vi "Generate Z stage Position Aarray.vi"(5 "Save PSOCT?":bool[](array[boolean]), 7 "#cycles":u32, 8 "Error in":errorcluster, 9 "Pause?":bool[](array[boolean]), 10 "image thickness":u32[](array[numeric]), 11 "slice thickness":u32[](array[numeric])) -> (0 "Error out":errorcluster, 1 "Cut Pauser":bool[](array[boolean]), 2 "image height out":dbl[](array[numeric]), 3 "cut height out":dbl[](array[numeric]), 4 "Save PSOCT?":bool[](array[boolean]))   [LabVIEW 2018]
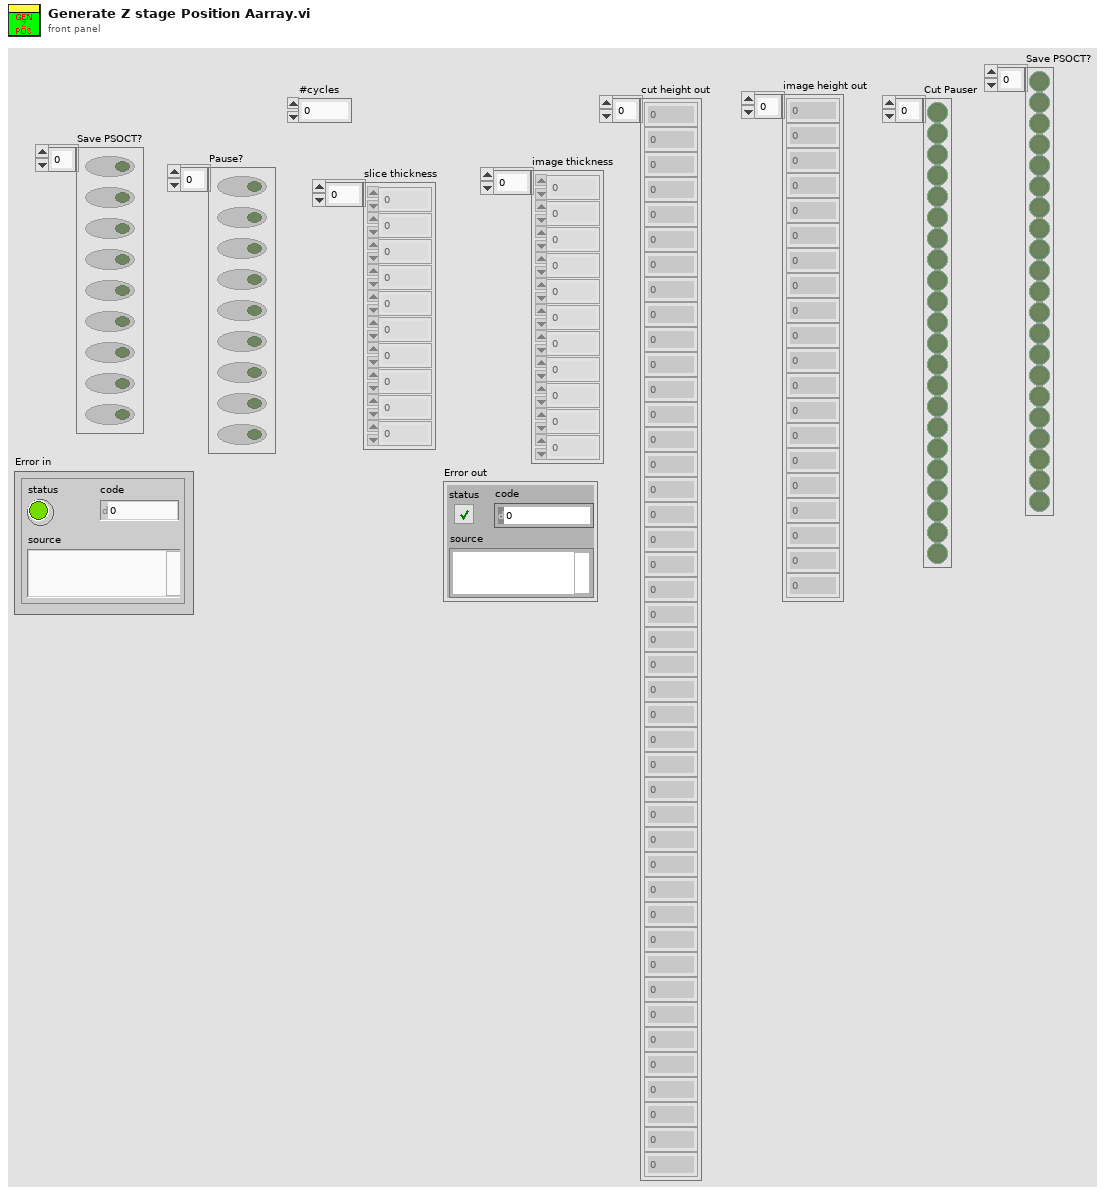
[diagram p1: front panel]
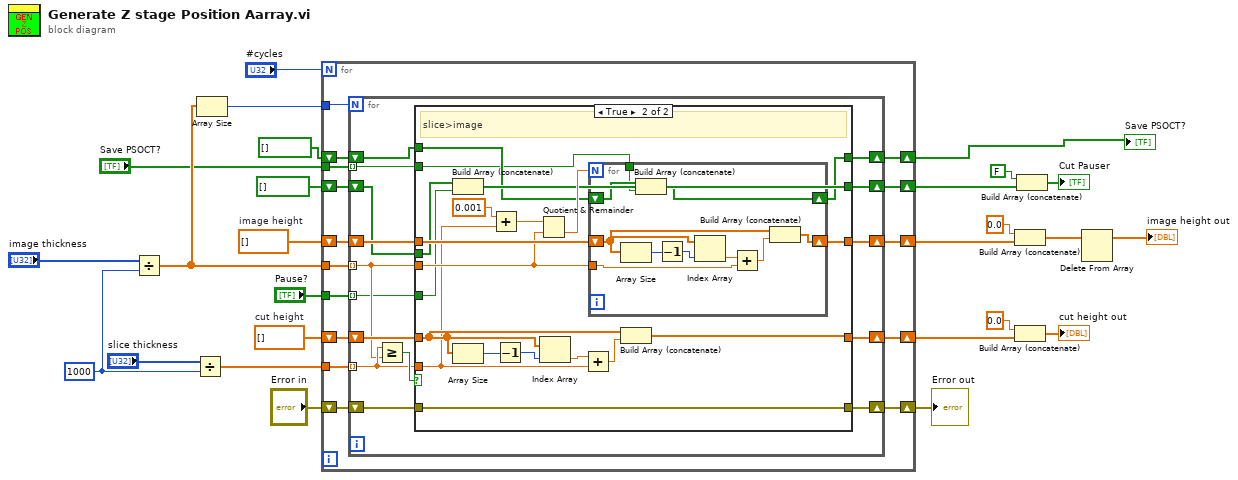
[diagram p0: block diagram]
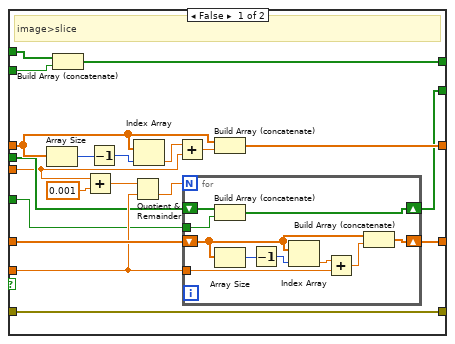
[diagram p2: hidden frame]
diagram:
  w21 = dbl[] []  # image height
  w26 = 1000
  w22 = dbl[] []  # cut height
  n1 = Divide(x="image thickness", y=w26) -> (x/y=w7:dbl[])
  n2 = Divide(x="slice thickness", y=w26) -> (x/y=w6:dbl[])
  n3 = Array Size(array=w7) -> (size(s)=w4:i32)
  n4 = for {
    N: "#cycles" -> [_]
    shift-right: [w36] -> w19
    shift-left: w22 -> [w41]
    tunnel: w6 -> [w40]
    tunnel: w7 -> [w39]
    tunnel: w4 -> [w35]
    shift-right: [w37] -> w16
    shift-left: w21 -> [w38]
    tunnel: "Pause?" -> [w33]
    shift-right: [w32] -> w11
    shift-left: bool[] [] -> [w34]
    shift-right: [w30] -> w8
    shift-left: "Error in" -> [w31]
    tunnel: "Save PSOCT?" -> [w29]
    shift-right: [w27] -> w1
    shift-left: bool[] [] -> [w28]
    n5 = for {
      N: w35 -> [_]
      shift-right: [w54] -> w36
      shift-left: w41 -> [w56]
      tunnel: w40 -> [w51] mode=indexing
      tunnel: w39 -> [w50] mode=indexing
      shift-right: [w53] -> w37
      shift-left: w38 -> [w55]
      tunnel: w33 -> [w48] mode=indexing
      shift-right: [w47] -> w32
      shift-left: w34 -> [w49]
      shift-right: [w45] -> w30
      shift-left: w31 -> [w46]
      tunnel: w29 -> [w44] mode=indexing
      shift-right: [w42] -> w27
      shift-left: w28 -> [w43]
      n6 = Greater Or Equal?(x=w51, y=w50) -> (x >= y?=w52:bool)
      n7 = case shown="True" w52 {
        tunnel: w56 -> [w73 w99]
        tunnel: w55 -> [w69 w102]
        tunnel: w51 -> [w72 w91]
        tunnel: [w71 w104] -> w54
        tunnel: w50 -> [w62 w100]
        tunnel: [w70 w101] -> w53
        tunnel: w49 -> [w66 w96]
        tunnel: w48 -> [w65 w95]
        tunnel: [w64 w94] -> w47
        tunnel: w46 -> [w63 w93]
        tunnel: [w63 w93] -> w45
        tunnel: w44 -> [w58 w88]
        tunnel: w43 -> [w59 w89]
        tunnel: [w57 w87] -> w42
        frame False {
          # "image>slice"
          n8 = Array Size(array=w69) -> (size(s)=w67:i32)
          n9 = Build Array (concatenate)(w59, w58) -> (w57:bool[])
          n10 = Add(x=w62, y=0.001) -> (x+y=w60:dbl)
          n11 = Decrement(x=w67) -> (x-1=w68:i32)
          n12 = Quotient & Remainder(x=w60, y=w72) -> (floor(x/y)=w74:dbl)  [unwired: 1 out]
          n13 = Index Array(array=w69, index=w68) -> (element=w76:dbl)
          n14 = Add(x=w76, y=w62) -> (x+y=w75:dbl)
          n15 = for {
            N: w74 -> [_]
            tunnel: w72 -> [w85]
            shift-right: [w83] -> w71
            shift-left: w73 -> [w82]
            tunnel: w65 -> [w78]
            shift-right: [w77] -> w64
            shift-left: w66 -> [w79]
            n16 = Build Array (concatenate)(w79, w78) -> (w77:bool[])
            n17 = Array Size(array=w82) -> (size(s)=w81:i32)
            n18 = Decrement(x=w81) -> (x-1=w80:i32)
            n19 = Index Array(array=w82, index=w80) -> (element=w86:dbl)
            n20 = Add(x=w86, y=w85) -> (x+y=w84:dbl)
            n21 = Build Array (concatenate)(w82, w84) -> (w83:dbl[])
          }
          n22 = Build Array (concatenate)(w69, w75) -> (w70:dbl[])
        }
        frame True {
          # "slice>image"
          n23 = Build Array (concatenate)(w96, w95) -> (w94:bool[])
          n24 = Array Size(array=w99) -> (size(s)=w98:i32)
          n25 = Add(x=0.001, y=w91) -> (x+y=w92:dbl)
          n26 = Decrement(x=w98) -> (x-1=w97:i32)
          n27 = Quotient & Remainder(x=w92, y=w100) -> (floor(x/y)=w103:dbl)  [unwired: 1 out]
          n28 = Index Array(array=w99, index=w97) -> (element=w106:dbl)
          n29 = Add(x=w106, y=w91) -> (x+y=w105:dbl)
          n30 = for {
            N: w103 -> [_]
            tunnel: w100 -> [w115]
            shift-right: [w113] -> w101
            shift-left: w102 -> [w112]
            shift-right: [w107] -> w87
            shift-left: w89 -> [w109]
            tunnel: w88 -> [w108]
            n31 = Array Size(array=w112) -> (size(s)=w111:i32)
            n32 = Build Array (concatenate)(w109, w108) -> (w107:bool[])
            n33 = Decrement(x=w111) -> (x-1=w110:i32)
            n34 = Index Array(array=w112, index=w110) -> (element=w116:dbl)
            n35 = Add(x=w116, y=w115) -> (x+y=w114:dbl)
            n36 = Build Array (concatenate)(w112, w114) -> (w113:dbl[])
          }
          n37 = Build Array (concatenate)(w99, w105) -> (w104:dbl[])
        }
      }
    }
  }
  "Error out" <- w8
  "Save PSOCT?" <- w1
  n38 = Build Array (concatenate)(0.0 ("element"), w16) -> (w15:dbl[])
  n39 = Build Array (concatenate)(0.0 ("element"), w19) -> (→"cut height out":dbl[])
  n40 = Build Array (concatenate)(FALSE ("Boolean"), w11) -> (→"Cut Pauser":bool[])
  n41 = Delete From Array(array=w15) -> (array with subset deleted=→"image height out":dbl[])  [unwired: 2 in, 1 out]
